vi "Axis_Init&Go_complex.vi"() -> ()   [LabVIEW 2020]
uses:
  <vilib>/Utility/error.llb/DialogType.ctl
panel:
  out "Index":i32=1 min=1 max=10
  in  "set vel":bool
  in  "Velocity":dbl format="%.3f"
  in  "stop":bool
  out "axis moving":bool
  in  "set mode":bool
  in  "start":bool
  in  "exit":bool
  in  "Target mode":u32(ring) items=["relative", "absolute", "NDT", "PT30", "free", ""]
  in  "Target":dbl format="%.3f"
  out "Axis position":dbl format="%.3f"
  in  "Axis number":i32=1 min=1 max=3
  in  "Control unit ID":i32=1 min=1 max=10
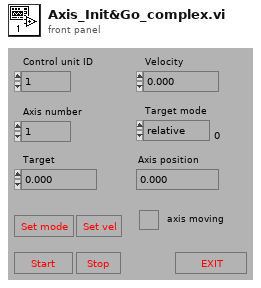
[diagram p1: front panel]
types:
  T1 = typedef "DialogType.ctl" = u16
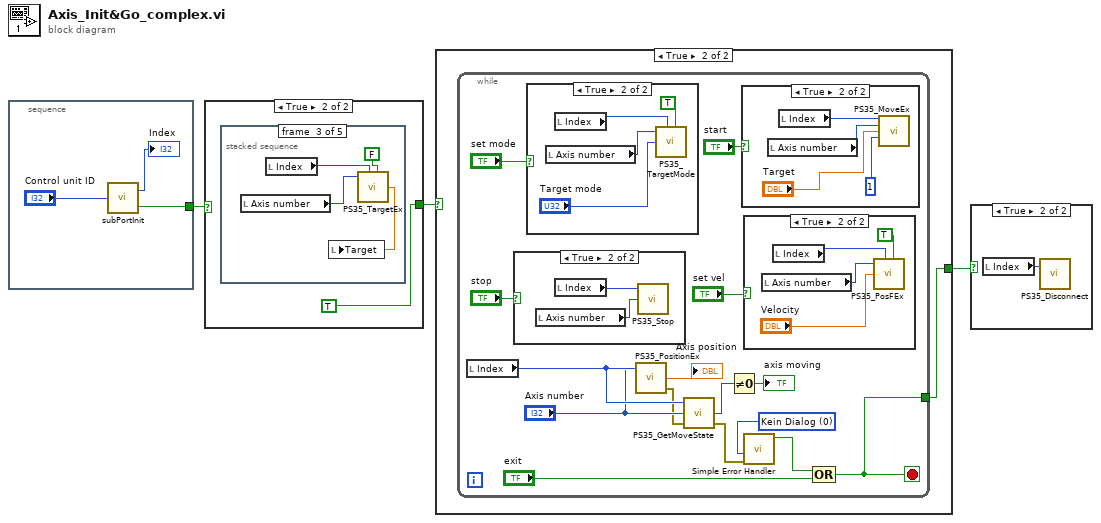
[diagram p0: block diagram]
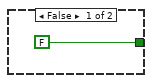
[diagram p2: hidden frame]
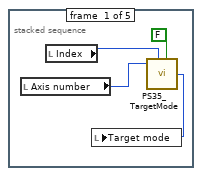
[diagram p3: hidden frame]
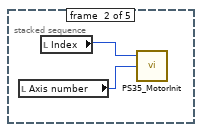
[diagram p4: hidden frame]
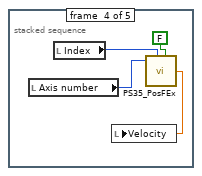
[diagram p5: hidden frame]
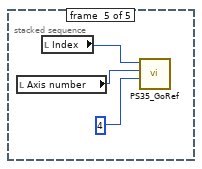
[diagram p6: hidden frame]
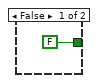
[diagram p8: hidden frame]
diagram:
  n1 = stacked-sequence {
    tunnel: [w6] -> w1
    frame #0 {
      n2 = call "subPortInit.vi"("Control unit ID"="Control unit ID") -> ("Index"=→"Index":i32, "InitOK"=w6:bool)
    }
  }
  n3 = case shown="True" w1 {
    tunnel: [FALSE ("function") TRUE ("function")] -> w2
    frame False {
    }
    frame True {
      n4 = stacked-sequence {
        frame #0 {
          n5 = local read "Axis number"() -> (w10:i32)
          n6 = local read "Index"() -> (w11:i32)
          n7 = call "PS35_TargetMode.vi"("Axis number"=w10, "Control unit ID"=w11, "function"=FALSE) -> ("Value-Out"=w9:i32)  [unwired: 5 in, 1 out]
          n8 = local write "Target mode"(w9) -> ()
        }
        frame #1 {
          n9 = local read "Axis number"() -> (w13:i32)
          n10 = local read "Index"() -> (w14:i32)
          n11 = call "PS35_MotorInit.vi"("Axis number"=w13, "Control unit ID"=w14) -> ()  [unwired: 2 in, 1 out]
        }
        frame #2 {
          n12 = local read "Axis number"() -> (w18:i32)
          n13 = local read "Index"() -> (w17:i32)
          n14 = call "PS35_TargetEx.vi"("Axis number"=w18, "Control unit ID"=w17, "function"=FALSE) -> ("dValue-Out"=w15:dbl)  [unwired: 5 in, 1 out]
          n15 = local write "Target"(w15) -> ()
        }
        frame #3 {
          n16 = local read "Axis number"() -> (w22:i32)
          n17 = local read "Index"() -> (w21:i32)
          n18 = call "PS35_PosFEx.vi"("Axis number"=w22, "Control unit ID"=w21, "function"=FALSE) -> ("dValue-Out"=w19:dbl)  [unwired: 5 in, 1 out]
          n19 = local write "Velocity"(w19) -> ()
        }
        frame #4 {
          n20 = local read "Axis number"() -> (w24:i32)
          n21 = local read "Index"() -> (w25:i32)
          n22 = call "PS35_GoRef.vi"("Mode"=4 ("Axis number"), "Axis number"=w24, "Control unit ID"=w25) -> ()  [unwired: 4 in, 1 out]
        }
      }
    }
  }
  n23 = case shown="True" w2 {
    tunnel: [FALSE ("stop") w27] -> w3
    frame False {
    }
    frame True {
      n24 = while {
        tunnel: [w34] -> w27
        stop <- w34 stop-if-true
        w31 = T1 0 items=["Kein Dialog", "OK-Nachricht", "Dialog zum Fortsetzen oder Anhalten", "OK Nachricht + Warnungen", "Weiter/Stop + Warnung"] ("type of dialog (OK msg:1)")
        n25 = local read "Index"() -> (w39:i32)
        n26 = case shown="True" "stop" {
          frame False {
          }
          frame True {
            n27 = local read "Axis number"() -> (w47:i32)
            n28 = local read "Index"() -> (w48:i32)
            n29 = call "PS35_Stop.vi"("Axis number"=w47, "Control unit ID"=w48) -> ()  [unwired: 2 in, 1 out]
          }
        }
        n30 = case shown="True" "set mode" {
          frame False {
          }
          frame True {
            n31 = local read "Axis number"() -> (w51:i32)
            n32 = local read "Index"() -> (w50:i32)
            n33 = call "PS35_TargetMode.vi"("Axis number"=w51, "Control unit ID"=w50, "Value-In"="Target mode", "function"=TRUE) -> ()  [unwired: 4 in, 2 out]
          }
        }
        n34 = call "PS35_PositionEx.vi"("Axis number"="Axis number", "Control unit ID"=w39) -> ("dValue-Out"=→"Axis position":dbl, "error out"=w32:errorcluster)  [unwired: 6 in]
        n35 = call "PS35_GetMoveState.vi"("error in (no error)"=w32, "Axis number"="Axis number", "Control unit ID"=w39) -> ("error out"=w29:errorcluster, "Move state"=w30:i32)  [unwired: 1 in]
        n36 = Not Equal To 0?(x=w30) -> (x != 0?=→"axis moving":bool)
        n37 = case shown="True" "start" {
          frame False {
          }
          frame True {
            n38 = local read "Axis number"() -> (w55:i32)
            n39 = local read "Index"() -> (w56:i32)
            n40 = call "PS35_MoveEx.vi"("Control unit ID"=w56, "Axis number"=w55, "dValue"="Target", "nEx"=1 ("bEx")) -> ()  [unwired: 11 in, 1 out]
          }
        }
        n41 = case shown="True" "set vel" {
          frame False {
          }
          frame True {
            n42 = local read "Axis number"() -> (w46:i32)
            n43 = local read "Index"() -> (w45:i32)
            n44 = call "PS35_PosFEx.vi"("Axis number"=w46, "Control unit ID"=w45, "dValue-In"="Velocity", "function"=TRUE) -> ()  [unwired: 4 in, 2 out]
          }
        }
        n45 = call <vilib>:"Simple Error Handler.vi"("type of dialog (OK msg:1)"=w31, "error in (no error)"=w29) -> ("error?"=w28:bool)  [unwired: 3 in, 4 out]
        n46 = Compound Arithmetic op=OR(w28, "exit") -> (w34:bool)
      }
    }
  }
  n47 = case shown="True" w3 {
    frame False {
    }
    frame True {
      n48 = local read "Index"() -> (w57:i32)
      n49 = call "PS35_Disconnect.vi"("Control unit ID"=w57) -> ()  [unwired: 2 in, 1 out]
    }
  }
